vi "Fetch Multi Eval Meas IQ Absolute Trace Result.vi"(0 "VISA resource name":refnum<visa-resource-name>, 5 "Instance (1)":i32=1, 7 "Trace Type (Absolute)":i32(ring) items=["Absolute", "Offset"], 11 "error in (no error)":errorcluster) -> (4 "VISA resource name out":refnum<visa-resource-name>, 6 "Reliability":i32, 8 "I Phase":dbl[](array[numeric]) format="%^.3e", 10 "Q Phase":dbl[](array[numeric]) format="%^.3e", 15 "error out":errorcluster)   [LabVIEW 2015, in "Rohde&Schwarz CMP LR WPAN Measurement.lvlib"]
doc: "Returns the absolute I/Q constellation diagram (I/Q points at each chip interval within the PSDU are returned).\n\nReturn values:\n<Reliability> - Reliability indicator\n<I_1> <Q_1> ... <I_10240> <Q_10240> - Pairs of normalized I and Q amplitudes\n\nAttribute:\n-\n\nRemote-control commands:\nFETCh:WPAN:MEAS<i>:MEValuation:TRACe:IQABsolute?\nFETCh:WPAN:MEAS<i>:MEValuation:TRACe:IQOFfset?"
uses:
  <instrlib>/Rohde&Schwarz CMP LR WPAN Measurement/Rohde&Schwarz CMP LR WPAN Measurement.lvlib
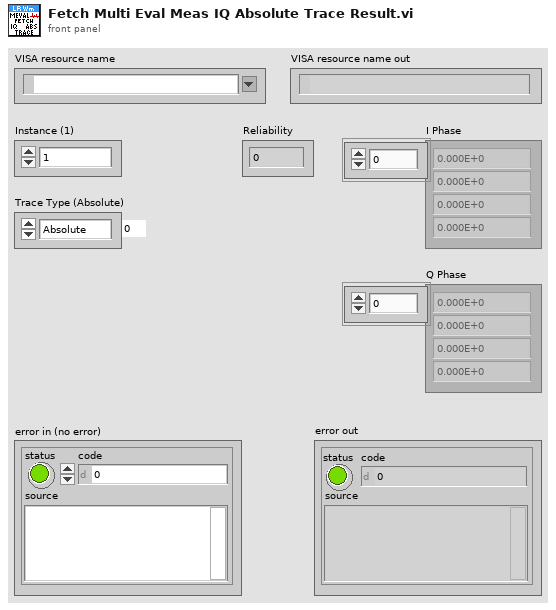
[diagram p1: front panel]
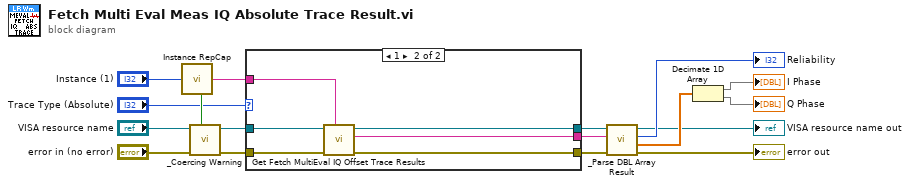
[diagram p0: block diagram]
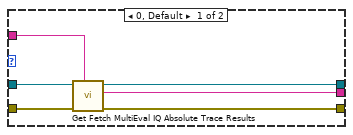
[diagram p2: hidden frame]
diagram:
  n1 = call <instrlib>:"Instance RepCap.vi"("Instance In"="Instance (1)") -> ("In Range?"=w17:bool, "RepCap Identifier Out"=w16:string)  [unwired: 1 in]
  n2 = call <instrlib>:"_Coercing Warning.vi"("In Range?"=w17, "error in (no error)"="error in (no error)", "VISA resource name"="VISA resource name") -> ("error out"=w13:errorcluster, "VISA resource name out"=w12:refnum<visa-resource-name>)  [unwired: 7 in]
  n3 = case shown="1" "Trace Type (Absolute)" {
    tunnel: w12 -> [w21 w29]
    tunnel: w13 -> [w22 w28]
    tunnel: w16 -> [w23 w27]
    tunnel: [w20 w26] -> w4
    tunnel: [w19 w25] -> w3
    tunnel: [w18 w24] -> w2
    frame 0, Default {
      n4 = call "Get Fetch MultiEval IQ Absolute Trace Results"("Repeated Capabilities"=w23, "error in (no error)"=w22, "instrument handle"=w21) -> ("error out"=w19:errorcluster, "Fetch MultiEval IQ Absolute Trace Results"=w18:string, "instrument handle out"=w20:refnum<visa-resource-name>)  [unwired: 6 in]
    }
    frame 1 {
      n5 = call "Get Fetch MultiEval IQ Offset Trace Results"("Repeated Capabilities"=w27, "error in (no error)"=w28, "instrument handle"=w29) -> ("error out"=w25:errorcluster, "Fetch MultiEval IQ Offset Trace Results"=w24:string, "instrument handle out"=w26:refnum<visa-resource-name>)  [unwired: 6 in]
    }
  }
  n6 = call <instrlib>:"_Parse DBL Array Result.vi"("error in (no error)"=w3, "Input String"=w2, "VISA resource name"=w4) -> ("error out"=→"error out":errorcluster, "Results"=w8:dbl[], "Reliability"=→"Reliability":i32, "VISA resource name out"=→"VISA resource name out":refnum<visa-resource-name>)  [unwired: 5 in]
  n7 = Decimate 1D Array(w8) -> (→"I Phase":dbl[], →"Q Phase":dbl[])
